vi "Write Position.vi"(8 "error in (no error)":errorcluster, 10 "Coordinate":T1, 11 "GameMenu in":refnum<class "GameMenu.lvclass">) -> (0 "error out":errorcluster, 3 "GameMenu out":refnum<class "GameMenu.lvclass">)   [LabVIEW 2019, in "RT_Game.lvlib" / "GameMenu.lvclass"]
uses:
  GameMenu.lvclass
  Game/Coordinate.ctl
  GameMenu.lvclass/GameMenu.ctl
  Game/Game.lvclass
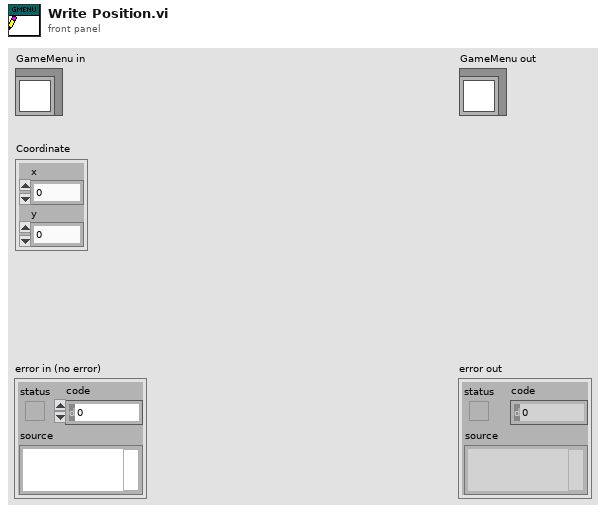
[diagram p1: front panel]
types:
  T1 = typedef "RT_Game.lvlib/Game.lvclass/Coordinate.ctl" = cluster{"x":dbl, "y":dbl}
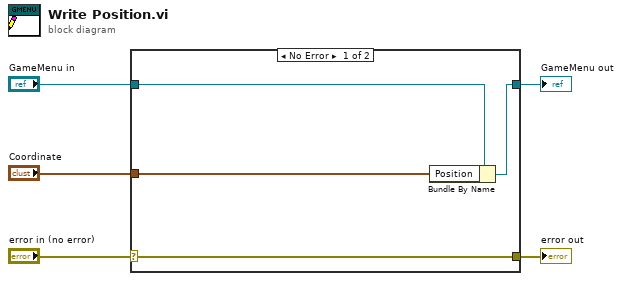
[diagram p0: block diagram]
diagram:
  n1 = case shown="No Error" "error in (no error)" {
    selector: "error in (no error)" -> [w9 w10]
    tunnel: [w9 w10] -> w4
    tunnel: [w7 w11] -> w2
    tunnel: "GameMenu in" -> [w8 w11]
    tunnel: "Coordinate" -> [w6 _]
    frame No Error {
      n2 = Bundle By Name(cluster=w8, "Position"=w6) -> (w7:refnum<class "GameMenu.lvclass">)
    }
    frame Error {
    }
  }
  "error out" <- w4
  "GameMenu out" <- w2
